vi "Topics Strings--constant.vi"() -> (3 "Topics Strings":string[](array[string]))   [LabVIEW 2016, in "MQTT_Client.lvlib"]
uses:
  MQTT_Client.lvlib
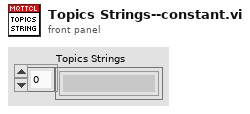
[diagram p1: front panel]
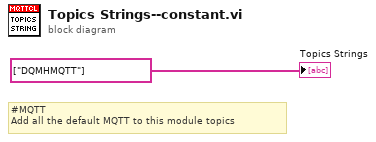
[diagram p0: block diagram]
diagram:
  # "#MQTT   \nAdd all the default MQTT to this module topics"
  "Topics Strings" <- string[] ["DQMHMQTT"]
